vi "(SubVI) Sliding-Window Average Filters_YCC.vi"(4 "All add in the tail?":bool, 5 "Avg points":i32, 7 "Signal":dbl[](array[numeric])) -> (3 "Filtered Signal":dbl[](array[numeric]))   [LabVIEW 2014]
uses:
  <vilib>/Analysis/baseanly.llb/Mean (DBL).vi
  <vilib>/Analysis/NI_AALBase.lvlib
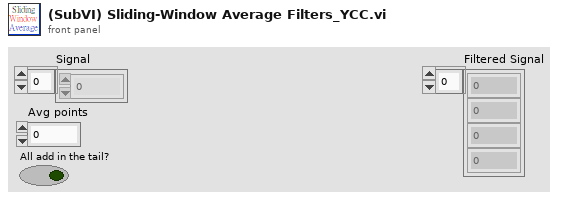
[diagram p1: front panel]
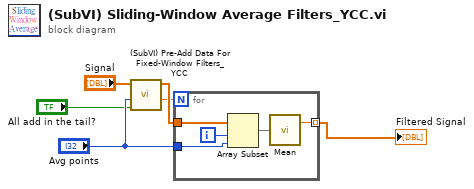
[diagram p0: block diagram]
diagram:
  n1 = call "(SubVI) Pre-Add Data For Fixed-Window Filters_YCC.vi"("All add in the tail?"="All add in the tail?", "Avg points"="Avg points", "Signal"="Signal") -> ("loop # for Silding window"=w3:dbl, "added-Signal"=w4:dbl[])  [unwired: 3 in]
  n2 = for {
    N: w3 -> [_]
    tunnel: w4 -> [w11]
    tunnel: "Avg points" -> [w8]
    tunnel: [w9] -> w2 mode=indexing
    i -> [w7]
    n3 = Array Subset(array=w11, index=w7, length=w8) -> (w10:dbl[])
    n4 = call-poly <vilib>:"Mean.vi"("X"=w10) -> ("mean"=w9:dbl)  [unwired: 1 out]
  }
  "Filtered Signal" <- w2
